vi "Read MonoCommunicator.vi"(8 "error in (no error)":errorcluster, 11 "Monochromator in":refnum<class "Monochromator.lvclass">) -> (0 "error out":errorcluster, 2 "MonoCommunicator.lvclass":refnum<class "MonoCommunicator.lvclass">, 3 "Monochromator out":refnum<class "Monochromator.lvclass">)   [LabVIEW 2016, in "Monochromator.lvclass"]
uses:
  Monochromator.lvclass
  MonoCommunicator/MonoCommunicator.lvclass
  Monochromator.lvclass/Monochromator.ctl
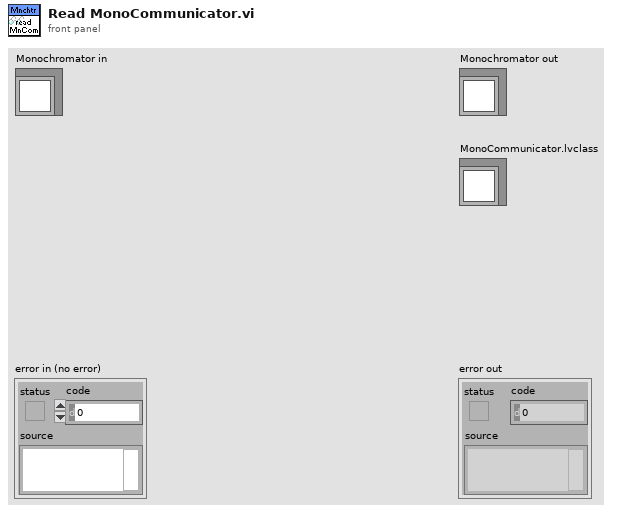
[diagram p1: front panel]
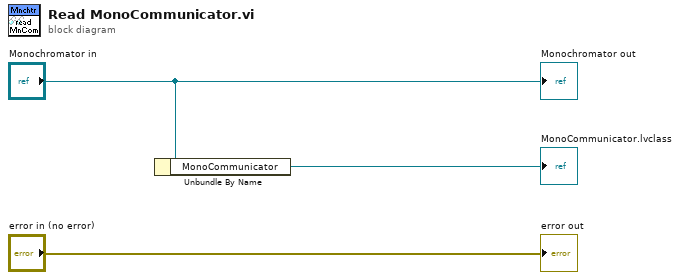
[diagram p0: block diagram]
diagram:
  n1 = Unbundle By Name("Monochromator in") -> ("MonoCommunicator"=→"MonoCommunicator.lvclass":refnum<class "MonoCommunicator.lvclass">)
  "error out" <- "error in (no error)"
  "Monochromator out" <- "Monochromator in"
